vi "LuaVIEW Push (path).vi"(0 "path":path, 5 "LuaVIEW reference in":T1, 11 "error in (no error)":errorcluster) -> (6 "LuaVIEW reference out":T1, 15 "error out":errorcluster)   [LabVIEW 2013]
doc: "Converts a path into a string and pushes that string onto the Lua stack. The conversion performed is identical to LabVIEW's \"Path to String\" conversion function. This VI is part of a polymorphic set that supports various data types. To change the type being pushed, pop up on this VI's diagram icon and use the \"Select Type\" sub menu. When \"automatic\" is checked in that menu, wiring a different type to the top left input will cause the appropriate VI to be selected automatically."
uses:
  typedefs/t_LuaVIEW Reference.ctl
  typedefs/et_LuaVIEW CIN Actions.ctl
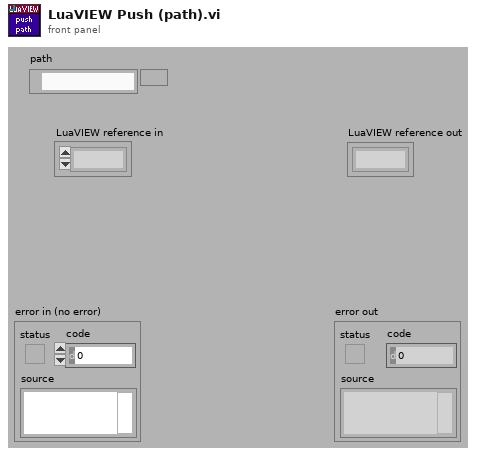
[diagram p1: front panel]
types:
  T1 = typedef "t_LuaVIEW Reference.ctl" = refnum<k1>
  T2 = typedef "et_LuaVIEW CIN Actions.ctl" = enum16{"checksynopsis", "_open", "_registerpublic", "_registerexport", "__never_an_error_result_ns", "luaversion", "cinversion", "_totals", "_taskcount", "pathological", "_unregnextpublic", "registryusecount", "__per_state_actions", "regsetprivate", "regsetindex", "regsetmodule", "_revokeexports", "_usepublic", "prepare", "compile", "execute", "call", "unregstaterefs", "_close", "pullboolean", "pullnumber", "pullI8", "pullU8", "pullI16", "pullU16", "pullI32", "pullU32", "pullobject", "pullrefnum", "pullstring", "pullflat", "pushflat", "pushobject", "getattribute", "setattribute", "stacktostring", "_startyieldtest", "_endyieldtest", "_pollprintbuffer", "__never_an_error_result_ps", "_pollexport", "setclone", "forcecleanup", "gettop", "clearstack", "insert", "pushboolean", "pushnumber", "pushrefnum", "pushstring", "pushnil", "pushvalue", "gettaskref", "settaskref"}
  T3 = typedef "et_LuaVIEW CIN Results.ctl" = enum16{"OK", "error", "main", "call", "clonecall", "modulecall", "exportcall", "index", "yield"}
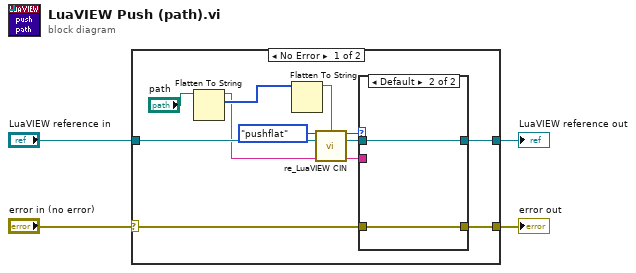
[diagram p0: block diagram]
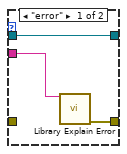
[diagram p2: hidden frame]
diagram:
  n1 = case shown="No Error" "error in (no error)" {
    selector: "error in (no error)" -> [w8 w23]
    tunnel: [w7 w22] -> w4
    tunnel: [w9 w23] -> w3
    tunnel: "LuaVIEW reference in" -> [w6 w22]
    frame No Error {
      n2 = Flatten To String(anything="path") -> (data string=w5:string, type string=w10:i16[])  [unwired: 3 in, 1 out]
      n3 = Flatten To String(anything=w10) -> (data string=w11:string)  [unwired: 3 in, 2 out]
      n4 = call "re_LuaVIEW CIN.vi"("action"=et_LuaVIEW_CIN_Actions."pushflat", "supplement"=w11, "LuaVIEW reference in"=w6, "string in"=w5) -> ("result"=w13:T3, "LuaVIEW reference out"=w14:T1, "string out"=w12:string)  [unwired: 5 in, 4 out]
      n5 = case shown="Default" w13 {
        tunnel: w14 -> [w17 w20]
        tunnel: [w17 w20] -> w7
        tunnel: [w19 w21] -> w9
        tunnel: w12 -> [w18 _]
        tunnel: w8 -> [_ w21]
        frame "error" {
          n6 = call "Library Explain Error.vi"("explanation prefix (none)"=w18) -> ("explained error"=w19:errorcluster)  [unwired: 14 in]
        }
        frame Default {
        }
      }
    }
    frame Error {
    }
  }
  "LuaVIEW reference out" <- w4
  "error out" <- w3
